vi "trabalho_cluster.vi"() -> ()   [LabVIEW 2020]
uses:
  <vilib>/addons/control/pid/pid.llb/PID Advanced (DBL).vi
  <vilib>/addons/control/pid/NI_PID_pid.lvlib
panel:
  in  "Controle numerico":dbl
  in  "LED IN":bool
  out "Novo":T1
  in  "stop":bool
  in  "Original":T2
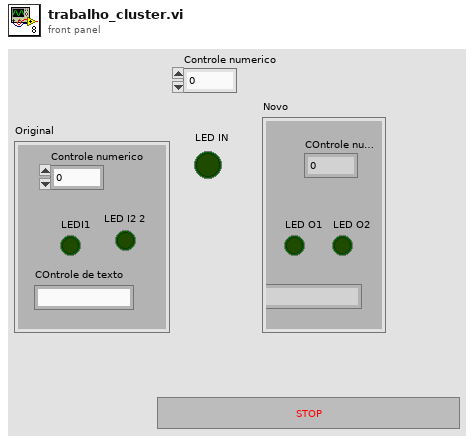
[diagram p1: front panel]
types:
  T1 = cluster{"COntrole numerico":dbl, "LED O1":bool, "LED O2":bool, "Controle de texto":string}
  T2 = cluster{"Controle numerico":dbl, "LEDI1":bool, "LED I2 2":bool, "COntrole de texto":string}
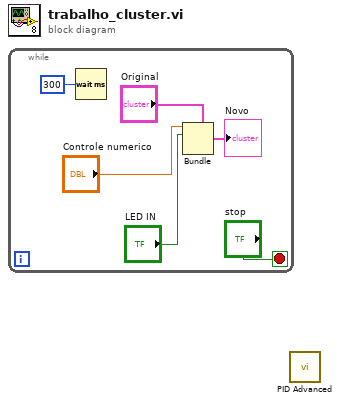
[diagram p0: block diagram]
diagram:
  n1 = while {
    stop <- "stop" stop-if-true
    n2 = Wait (ms)(milliseconds to wait=u32 300) -> ()  [unwired: 1 out]
    n3 = Bundle(cluster="Original", "Controle numerico"="Controle numerico", "LEDI1"="LED IN") -> (→"Novo":T2)  [unwired: 2 in]
  }
  n4 = call-poly <vilib>:"PID Advanced.vi"() -> ()  [unwired: 14 in, 2 out]
